vi "testUintSort.vi"(8 "error in (no error)":errorcluster, 11 "TestCase in":refnum<class "UnitTestUintClass.lvclass">) -> (0 "error out":errorcluster, 3 "TestCase out":refnum<class "UnitTestUintClass.lvclass">)   [LabVIEW 2011, in "UnitTestUintClass.lvclass"]
uses:
  UnitTestUintClass.lvclass
  UnitTestUintClass.lvclass/UnitTestUintClass.ctl
  <vilib>/addons/_JKI Toolkits/VI Tester/TestCase.llb/TestCase.lvclass
  UintClass/UintClass.lvclass
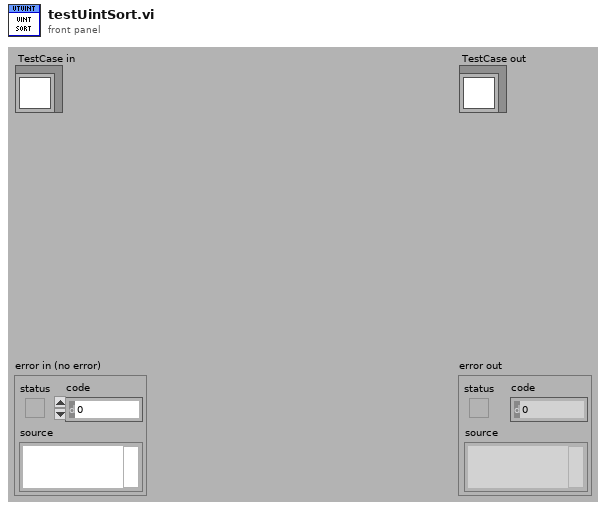
[diagram p1: front panel]
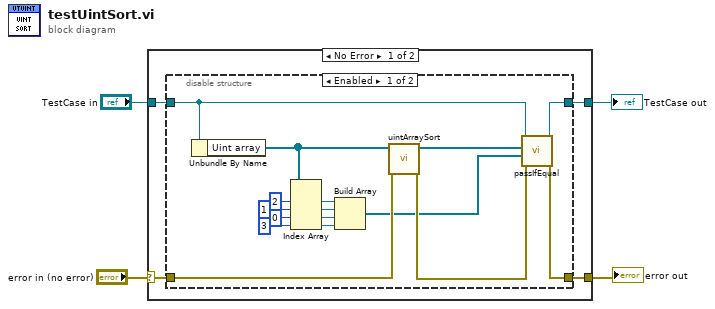
[diagram p0: block diagram]
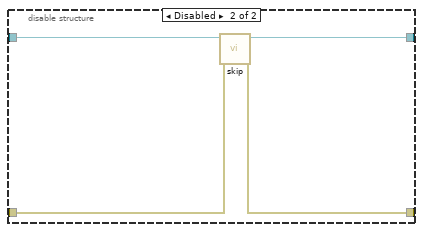
[diagram p2: hidden frame]
diagram:
  n1 = case shown="No Error" "error in (no error)" {
    selector: "error in (no error)" -> [w6 w30]
    tunnel: [w5 w30] -> w3
    tunnel: [w7 w29] -> w1
    tunnel: "TestCase in" -> [w8 w29]
    frame No Error {
      n2 = disable-structure shown="Enabled" {
        disable-tunnel: w8 -> [w22 w28]
        disable-tunnel: [w24 w25] -> w7
        disable-tunnel: w6 -> [w20 w27]
        disable-tunnel: [w23 w26] -> w5
        frame Enabled {
          n3 = Unbundle By Name(w22) -> ("Uint array"=w18:refnum<class "UintClass.lvclass">[])
          n4 = Index Array(array=w18, index #1=2 ("index"), index #2=1 ("index"), index #3=0 ("index"), index #4=3 ("index")) -> (element #1=w13:refnum<class "UintClass.lvclass">, element #2=w10:refnum<class "UintClass.lvclass">, element #3=w11:refnum<class "UintClass.lvclass">, element #4=w12:refnum<class "UintClass.lvclass">)
          n5 = Build Array(w13, w10, w11, w12) -> (w9:refnum<class "UintClass.lvclass">[])
          n6 = call "uintArraySort.vi"("Error in (no error)"=w20, "Uint array in"=w18) -> ("Error out"=w19:errorcluster, "Sorted uint array"=w21:refnum<class "UintClass.lvclass">[])  [unwired: 7 in, 1 out]
          n7 = call-dynamic "passIfEqual.vi"("error in (no error)"=w19, "y"=w9, "x"=w21, "TestCase in"=w22) -> ("error out"=w23:errorcluster, "TestCase out"=w24:refnum<class "UnitTestUintClass.lvclass">)  [unwired: 6 in]
        }
        frame Disabled {
          n8 = call <vilib>:"skip.vi"("error in (no error)"=w27, "TestCase in"=w28) -> ("error out"=w26:errorcluster, "TestCase out"=w25:refnum<class "UnitTestUintClass.lvclass">)  [unwired: 8 in]
        }
      }
    }
    frame Error {
    }
  }
  "error out" <- w3
  "TestCase out" <- w1
